vi "Set Or Get Num of Rows or Cols.vi"(6 "Row or Col Option":T1, 7 "Mode":T2, 8 "error in (no error)":errorcluster caption="错误输入（无错误）", 10 "Number of Rows or Cols In":u32, 11 "Table Ref In":refnum<vi>) -> (0 "error out":errorcluster caption="错误输出", 2 "Number of Rows or Cols Out":u32, 3 "Table Ref Out":refnum<vi>)   [LabVIEW 2013, in "Table Tool.lvlib"]
uses:
  Table Tool.lvlib
  Custum Type/GetOrSet.ctl
  Custum Type/Selet Row or Col.ctl
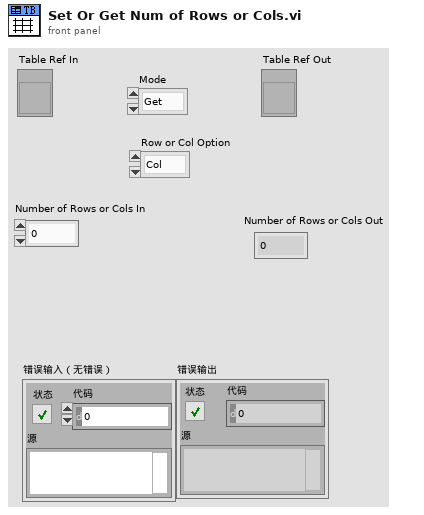
[diagram p1: front panel]
types:
  T1 = typedef "Table Tool.lvlib/Selet Row or Col.ctl" = enum16{"Col", "Row"}
  T2 = typedef "Table Tool.lvlib/GetOrSet.ctl" = enum16{"Get", "Set"}
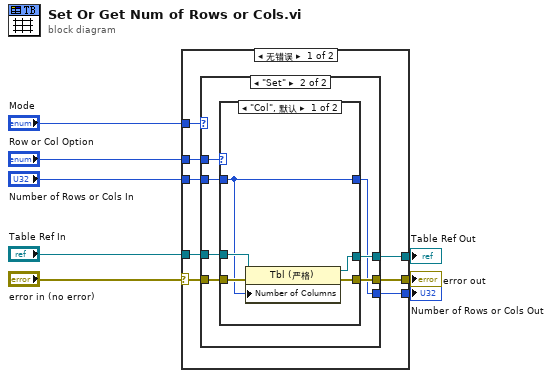
[diagram p0: block diagram]
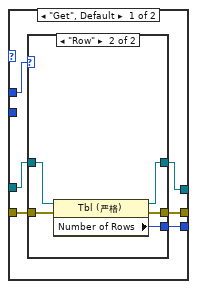
[diagram p2: hidden frame]
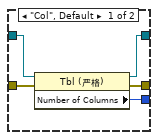
[diagram p3: hidden frame]
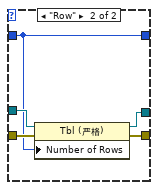
[diagram p4: hidden frame]
diagram:
  n1 = case shown="无错误" "error in (no error)" {
    selector: "error in (no error)" -> [w14 w51]
    tunnel: "Table Ref In" -> [w15 w50]
    tunnel: "Mode" -> [w16 _]
    tunnel: [w13 w50] -> w5
    tunnel: [w12 w51] -> w4
    tunnel: "Number of Rows or Cols In" -> [w11 _]
    tunnel: [w10 _] -> w2
    tunnel: "Row or Col Option" -> [w9 _]
    frame No Error {
      n2 = case shown="\"Set\"" w16 {
        tunnel: w15 -> [w21 w39]
        tunnel: w14 -> [w17 w38]
        tunnel: [w18 w37] -> w13
        tunnel: [w19 w36] -> w12
        tunnel: w11 -> [_ w35]
        tunnel: [w20 w33] -> w10
        tunnel: w9 -> [w22 w34]
        frame "Get", Default {
          n3 = case shown="\"Row\"" w22 {
            tunnel: w21 -> [w27 w31]
            tunnel: [w26 w30] -> w20
            tunnel: [w25 w28] -> w19
            tunnel: [w24 w29] -> w18
            tunnel: w17 -> [w23 w32]
            frame "Col", Default {
              n4 = property class="Tbl (严格)"(reference=w27, error in=w23) -> (reference out=w24:refnum<vi>, error out=w25:errorcluster, "Number of Columns"=w26:u32)
            }
            frame "Row" {
              n5 = property class="Tbl (严格)"(reference=w31, error in=w32) -> (reference out=w29:refnum<vi>, error out=w28:errorcluster, "Number of Rows"=w30:u32)
            }
          }
        }
        frame "Set" {
          n6 = case shown="\"Col\", 默认" w34 {
            tunnel: w39 -> [w44 w49]
            tunnel: w38 -> [w43 w48]
            tunnel: [w42 w47] -> w37
            tunnel: [w41 w46] -> w36
            tunnel: w35 -> [w40 w45]
            tunnel: [w40 w45] -> w33
            frame "Col", Default {
              n7 = property class="Tbl (严格)"(reference=w44, error in=w43, "Number of Columns"=w40) -> (reference out=w42:refnum<vi>, error out=w41:errorcluster)
            }
            frame "Row" {
              n8 = property class="Tbl (严格)"(reference=w49, error in=w48, "Number of Rows"=w45) -> (reference out=w47:refnum<vi>, error out=w46:errorcluster)
            }
          }
        }
      }
    }
    frame Error {
    }
  }
  "Table Ref Out" <- w5
  "error out" <- w4
  "Number of Rows or Cols Out" <- w2
